vi "Function.vi"(8 "error in (no error)":errorcluster, 9 "Bool B":T1, 10 "Bool A":T1, 11 "AND in":refnum<class "AND_I8.lvclass">) -> (0 "error out":errorcluster, 2 "Result":T1, 3 "AND out":refnum<class "AND_I8.lvclass">)   [LabVIEW 2021, in "AND_I8.lvclass"]
uses:
  AND_I8.lvclass
  Type.ctl
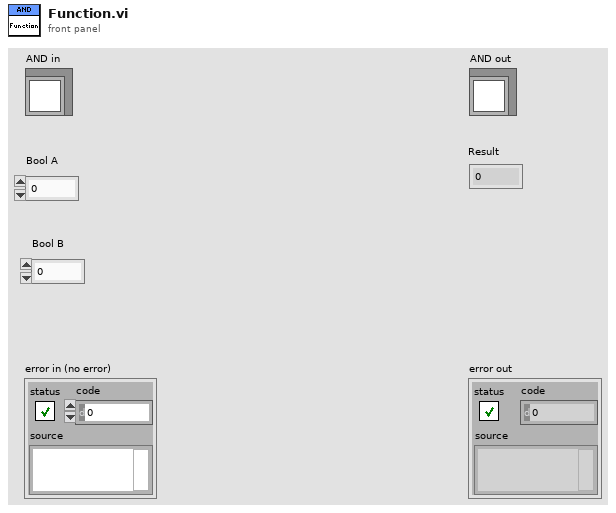
[diagram p1: front panel]
types:
  T1 = typedef "AND_I8.lvclass/Type.ctl" = i8
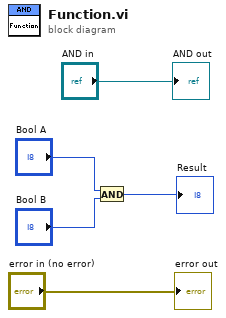
[diagram p0: block diagram]
diagram:
  n1 = And(x="Bool A", y="Bool B") -> (x .and. y?=→"Result":T1)
  "error out" <- "error in (no error)"
  "AND out" <- "AND in"
